vi "Ausgabe Diagramm.vi"() -> ()   [LabVIEW 2016]
doc: "Erstellen der Graphen und Anzeigen aller Parameter\n\nMöglichkeit zum Abspeichern des Graphen als PNG Format"
panel:
  in  "Array":i32[][](array[numeric])=[[5, 1], [4, 4], [3, 6], [4, 3], [2, 6], [4, 4], [7, 4], [3, 5], [2, 6], [1, 7]]
  in  "Array 3":i32[][](array[numeric])=[[0, 0], [1, 1], [2, 0], [3, 1], [4, 0], [-1, 1], [-2, 4], [-3, -5], [-4, 6], [-4, 7]]
  out "Namen":string
  out "Gruppe":string
  out "Probenbezeichnung":string
  out "Hmax [A/m]":dbl
  out "Bmax [T]":dbl
  out "Faktor 2":dbl
  out "Faktor 1":dbl
  out "Gwuenschte Frequenz [Hz]":dbl=15.0 min=15.0 max=15000.0 step=5.0
  out "Gewuenschte magn. Flussdichte [T]":dbl=0.001 min=0.001 max=5.0 step=0.001
  out "Messwiderstand [Ohm] 2":dbl=1.0 min=1.0 max=100.0
  out "Sekundaerwindungszahl 2":dbl=1.0 min=1.0 max=1500.0 step=1.0
  out "Primaerwindungszahl 2":dbl=1.0 min=1.0 max=1500.0 step=1.0
  out "Spannungsteilerverhaeltnis (1/x) 2":dbl=1.0 min=1.0 max=100.0 step=1.0
  out "Dichte des Eisens in [g/cm^3] 2":dbl=1.0 min=1.0 max=50.0 step=1.0
  out "Eisenquerschnitt A [mm^2] 2":dbl=1.0 min=1.0 max=10000.0 step=1.0
  out "Wirksame Laenge [cm] 2":dbl=94.0 min=0.0001 max=1000.0 step=0.5
  out "XY Graph":cluster{i32[], i32[]}[](graph)
  in  "Diagramm Speichern":bool
  in  "VI Speichern":bool
  out "Datum/Uhrzeit":timestamp
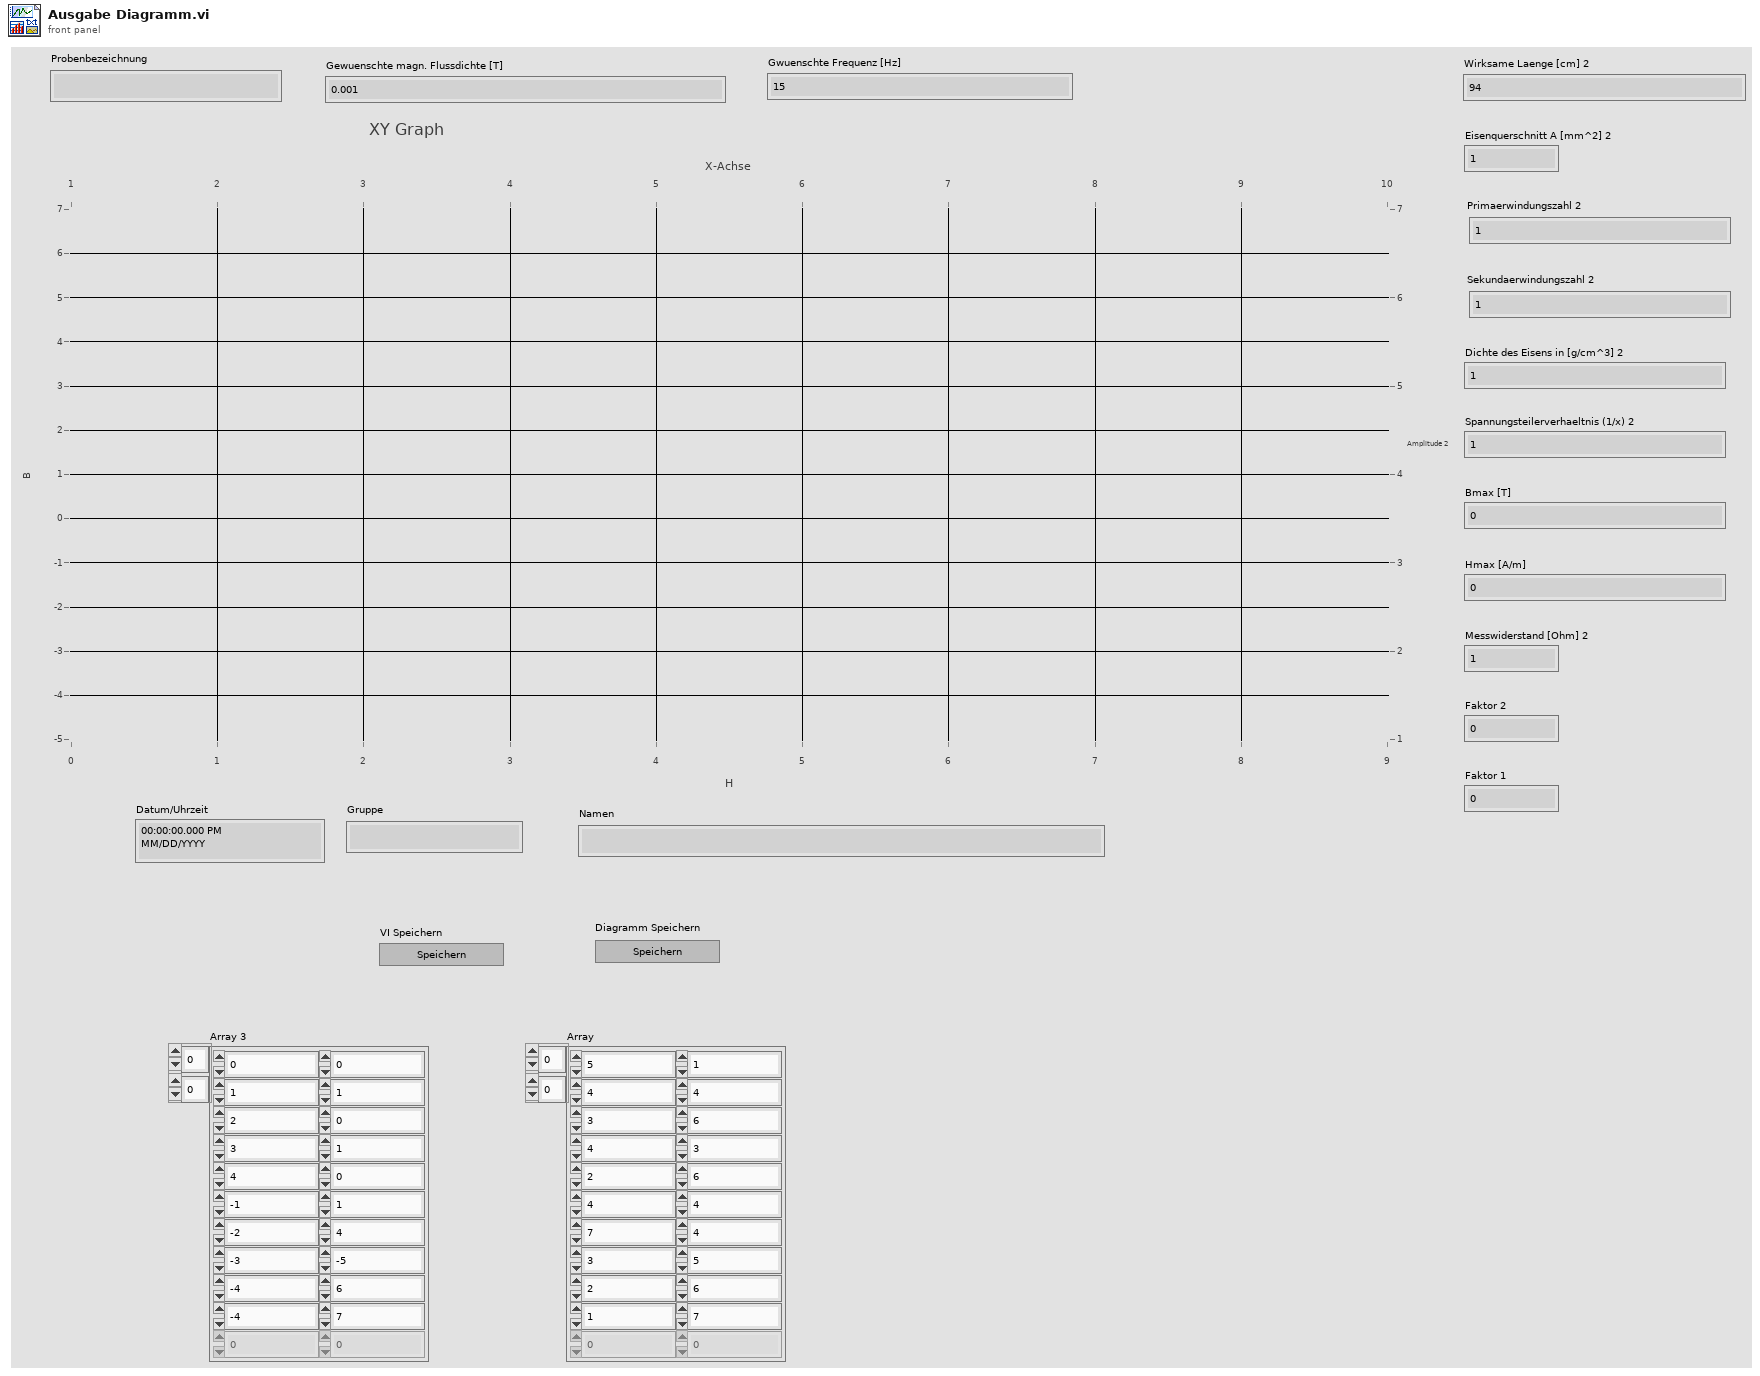
[diagram p1: front panel]
types:
  T1 = typedef "imagedata.ctl" = cluster{"image type":i32, "image depth":i32, "image":u8[], "mask":u8[], "colors":u32[], "Rectangle":cluster{"left":i16, "top":i16, "right":i16, "bottom":i16}}
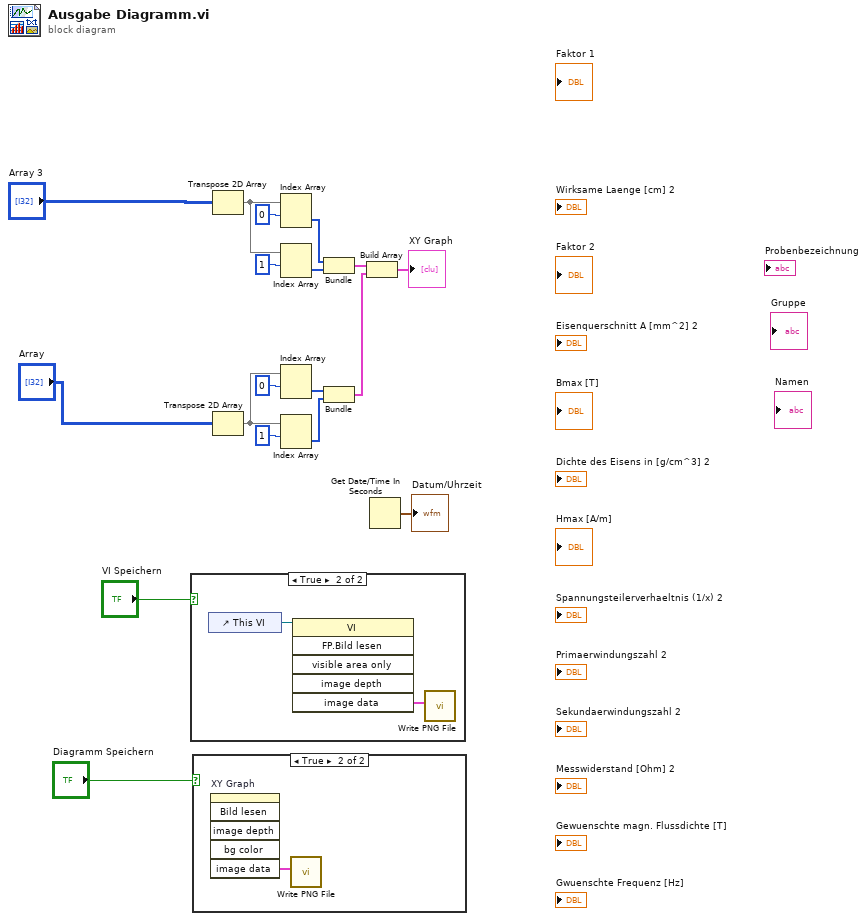
[diagram p0: block diagram]
diagram:
  n1 = case shown="True" "VI Speichern" {
    frame False {
    }
    frame True {
      n2 = control-ref of="This VI"() -> (w20:refnum<vi>)
      n3 = invoke class="VI" method="FP.Bild lesen"(reference=w20) -> ("image data"=w19:T1)  [unwired: 5 in, 5 out]
      n4 = call <vilib>:"Write PNG File.vi"("image data"=w19) -> ()  [unwired: 9 in, 2 out]
    }
  }
  n5 = case shown="True" "Diagramm Speichern" {
    frame False {
    }
    frame True {
      n6 = invoke on="XY Graph" class="XYGraph (strikt)" method="Bild lesen"() -> ("image data"=w21:T1)  [unwired: 6 in, 5 out]
      n7 = call <vilib>:"Write PNG File.vi"("image data"=w21) -> ()  [unwired: 9 in, 2 out]
    }
  }
  n8 = Transpose 2D Array(2D array="Array 3") -> (transposed array=w14:i32[][])
  n9 = Transpose 2D Array(2D array="Array") -> (transposed array=w4:i32[][])
  n10 = Index Array(array=w14, index (row)=0) -> (element=w12:i32[])  [unwired: 1 in]
  n11 = Index Array(array=w14, index (row)=1 ("Index (Zeile)")) -> (element=w11:i32[])  [unwired: 1 in]
  n12 = Index Array(array=w4, index (row)=0) -> (element=w7:i32[])  [unwired: 1 in]
  n13 = Index Array(array=w4, index (row)=1 ("Index (Zeile)")) -> (element=w6:i32[])  [unwired: 1 in]
  n14 = Bundle(w12, w11) -> (w3:cluster{i32[], i32[]})  [unwired: 1 in]
  n15 = Bundle(w7, w6) -> (w5:cluster{i32[], i32[]})  [unwired: 1 in]
  n16 = Build Array(w3, w5) -> (→"XY Graph":cluster{i32[], i32[]}[])
  n17 = Get Date/Time In Seconds() -> (seconds since 1Jan1904=→"Datum/Uhrzeit":timestamp)
